vi "GUI_PiezoControllerMMC-100.vi"() -> ()   [LabVIEW 2013]
doc: "Example of using standard HTTP protocol for recieving a web site (the HTML source)\n\n\nThis example uses the GET command. For general information about the HTTP protocol and other commands go to\nhttp://www.w3.org/Protocols\n\n\nBjornar Svingen\nbjornar.svingen@sintef.no bjornar.svingen@ktv.no"
uses:
  Shared/GUI_Template/GUI_master/tcp_new_data_event.ctl
  Shared/GUI_Template/GUI_master/tcp new data cluster.ctl
  <vilib>/Utility/config.llb/NI_LVConfig.lvlib
  <vilib>/Utility/config.llb/Read Key (String).vi
panel:
  in  "Axis polarity::1":enum16{"default", "inverted"}(ring) caption="Axis polarity"
  in  "Deceleration::1":dbl caption="Deceleration (mm/s^2)" min=0.0 max=500.0
  in  "Acceleration::1":dbl caption="Acceleration (mm/s^2)" min=0.0 max=500.0
  in  "Velocity::1":dbl caption="Velocity (mm/s)" min=0.0 max=100.0
  in  "Home::1":enum16{"HOME", "POS (+)", "NEG (-)", "done"}(ring) caption="Homing"
  in  "EnableMotor::1":bool caption="Motor enable"
  out "Motor status::1":T1(ring) caption="Motor status"
  in  "Nloop enable::1":bool caption="N-loop enable"
  out "Encoder position::1":dbl caption="Encoder pos. (mm)" min=-13.0 max=13.0 format="%.6f"
  in  "position::1":dbl caption="Position (mm)" min=-13.0 max=13.0 format="%.6f"
  out "tcp data event 2":T2
  out "GUIdevice 1":string="HeatTL1Stage"
  in  "Exit":bool
  out "Error":T3
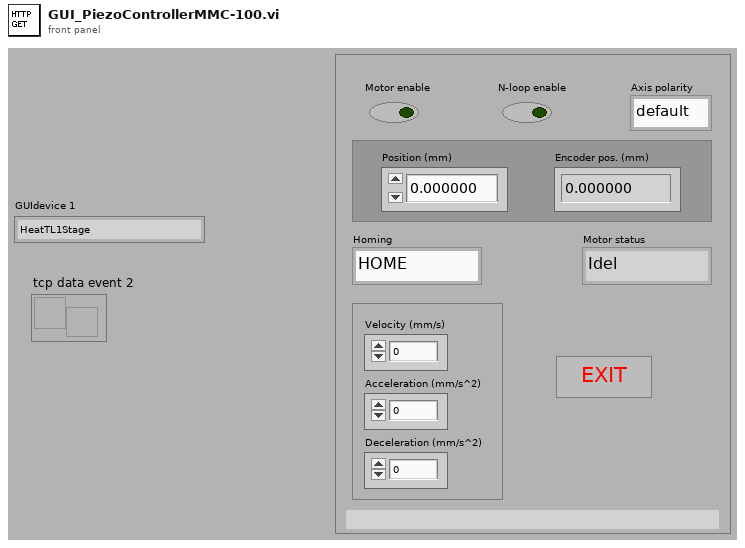
[diagram p1: front panel]
types:
  T1 = enum16{"Idel", "Moving", "Accelerating", "Decelerating", "L- (neg limit)", "L+ (pos limit)", "Homed", "Unknown"}
  T2 = typedef "tcp_new_data_event.ctl" = refnum<user-event>
  T3 = cluster{"status":bool, "code":i32, "UDP error message":string}
  T4 = enum32{"invalid app kind", "Development System", "Run Time System", "Student Edition", "Embedded LabVIEW", "Evaluation", "Custom"}
  T5 = typedef "tcp new data cluster.ctl" = cluster{"EventEnum":enum16{"new data", "connection status update"}, "Device name":string}
  T6 = enum32{"Invalid", "Standard", "Closed", "Hidden", "Minimized", "Maximized"}
  T7 = cluster{"Core":cluster{"Current VI Reference":refnum<vi>, "Close Panel on Exit?":bool}, "SuperGUI":cluster{"STOP queue":refnum<queue>, "SuperGUI ref":refnum<vi>, "event reg":refnum<event-registration>}, "Stage Device list":string[]}
  T8 = cluster{"STOP queue":refnum<queue>, "SuperGUI ref":refnum<vi>, "event reg":refnum<event-registration>}
  T9 = cluster{"Current VI Reference":refnum<vi>, "Close Panel on Exit?":bool}
  T10 = typedef "NI_LVConfig.lvlib/Config Data RefNum.ctl" = refnum<k1>
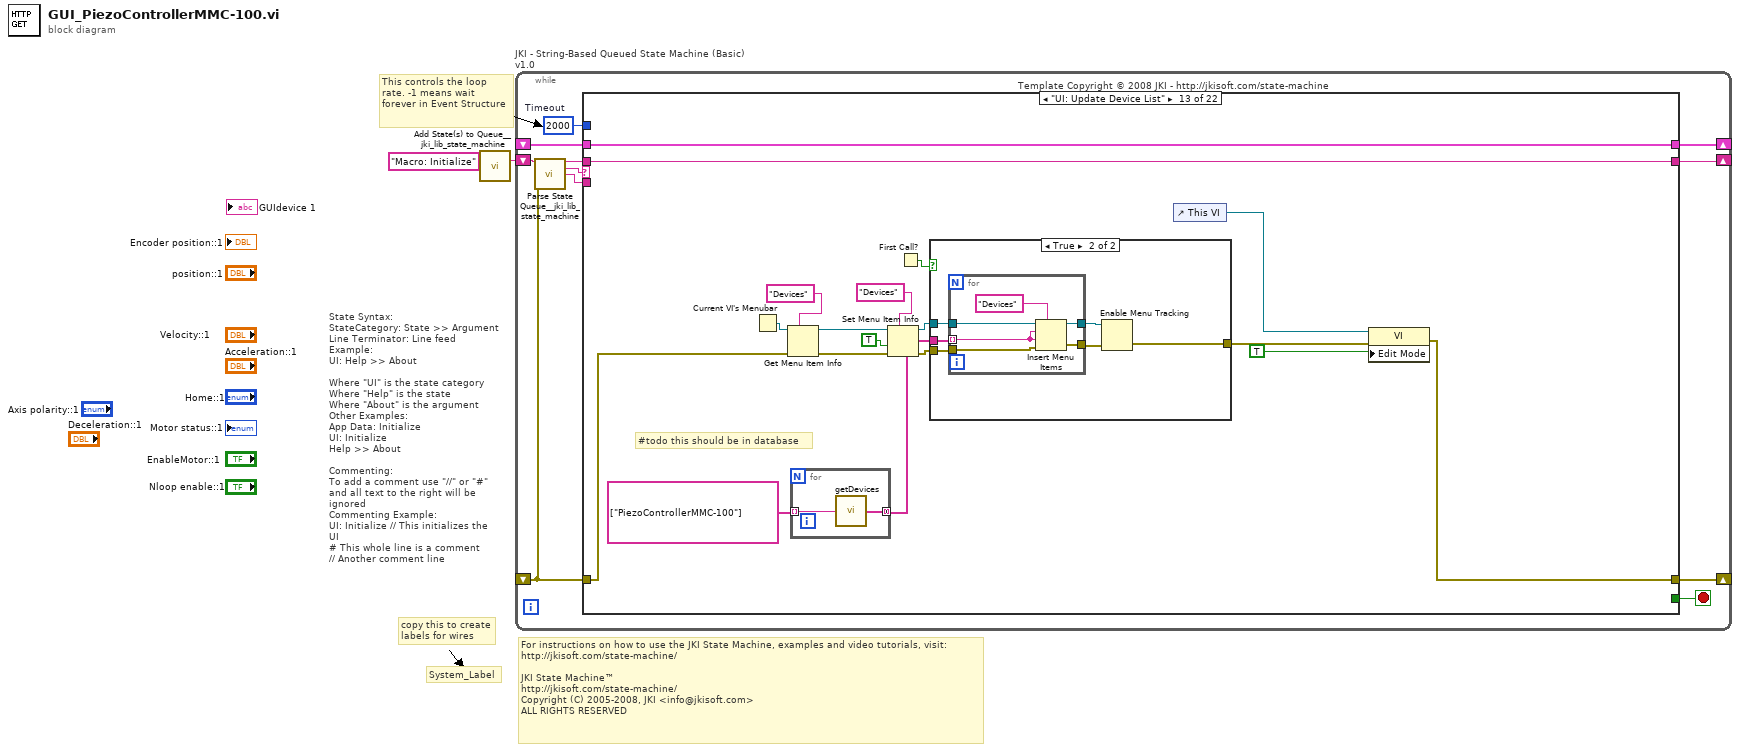
[diagram p0: block diagram]
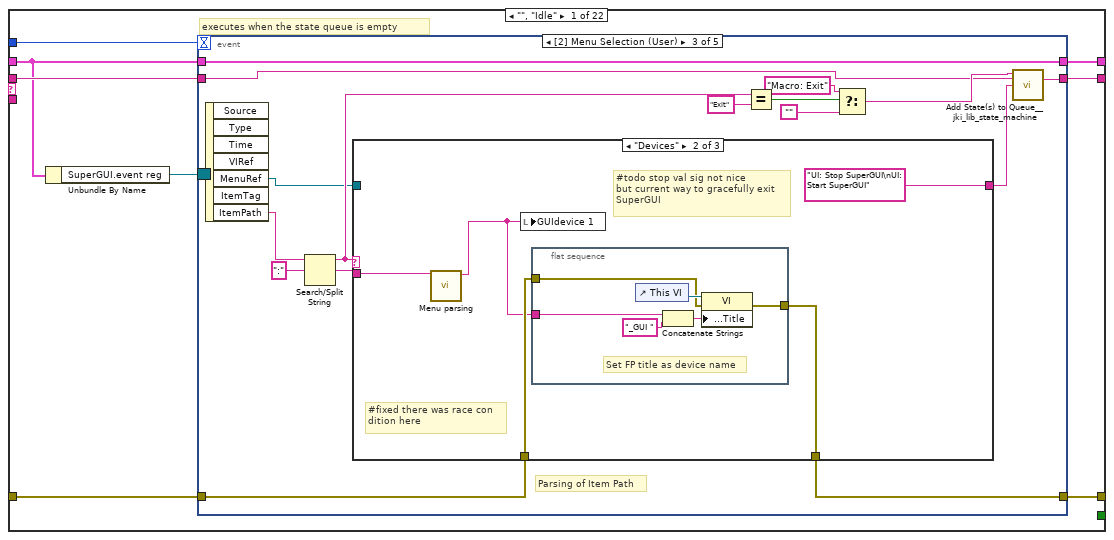
[diagram p2: hidden frame]
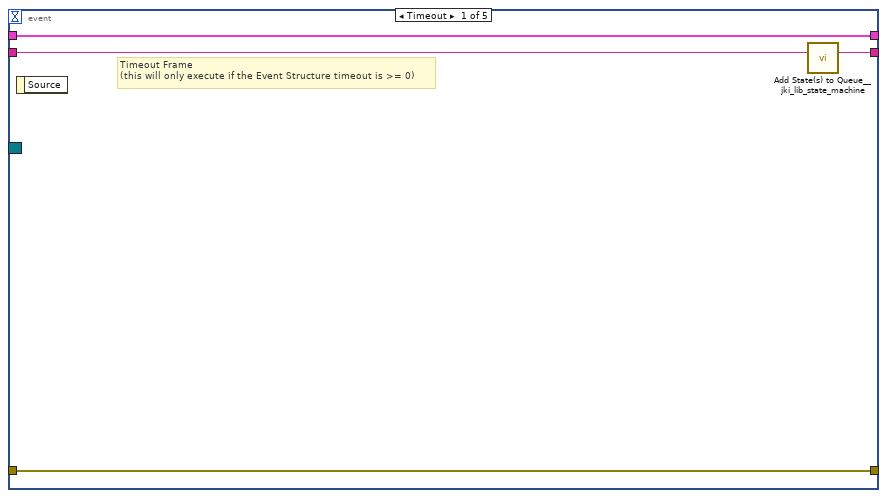
[diagram p3: hidden frame]
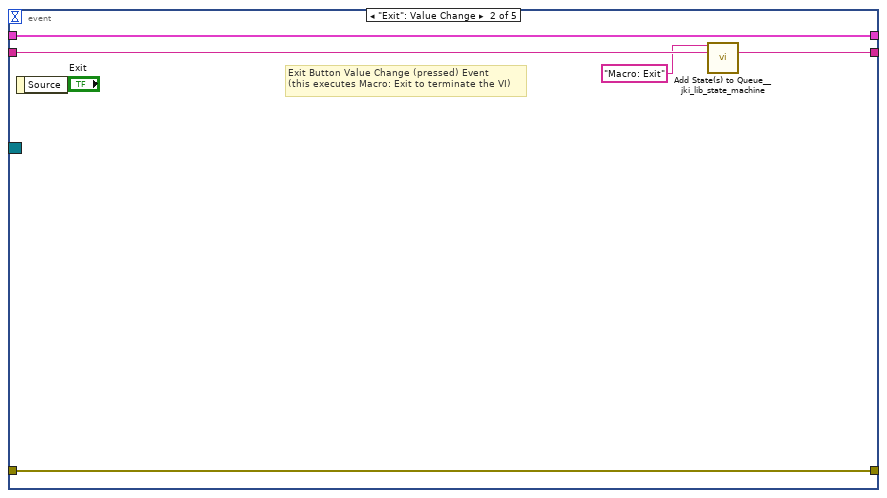
[diagram p4: hidden frame]
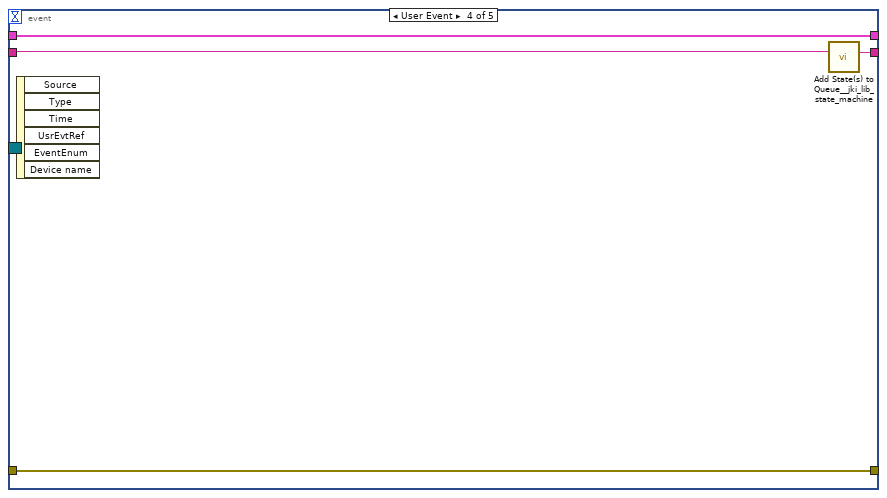
[diagram p7: hidden frame]
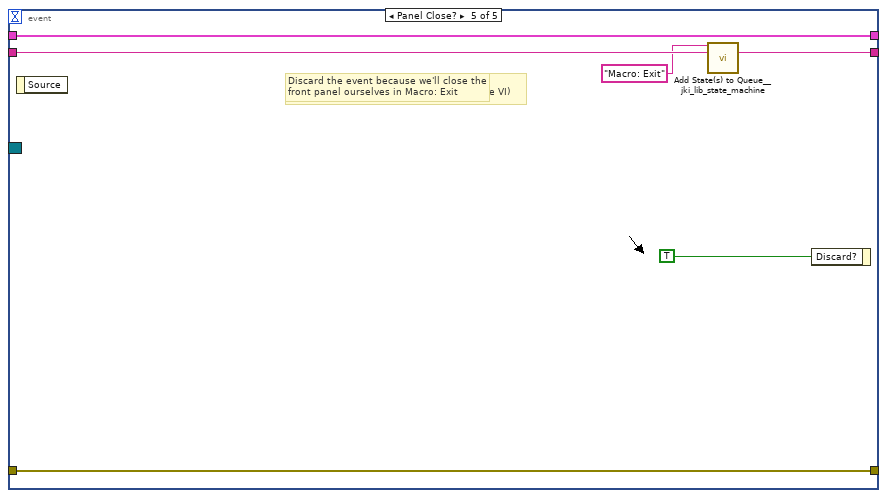
[diagram p8: hidden frame]
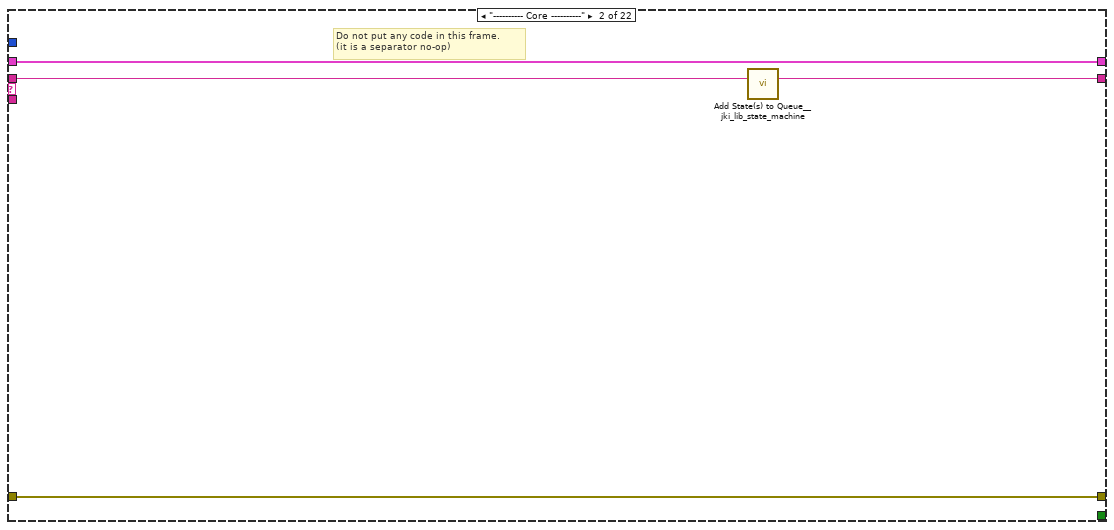
[diagram p9: hidden frame]
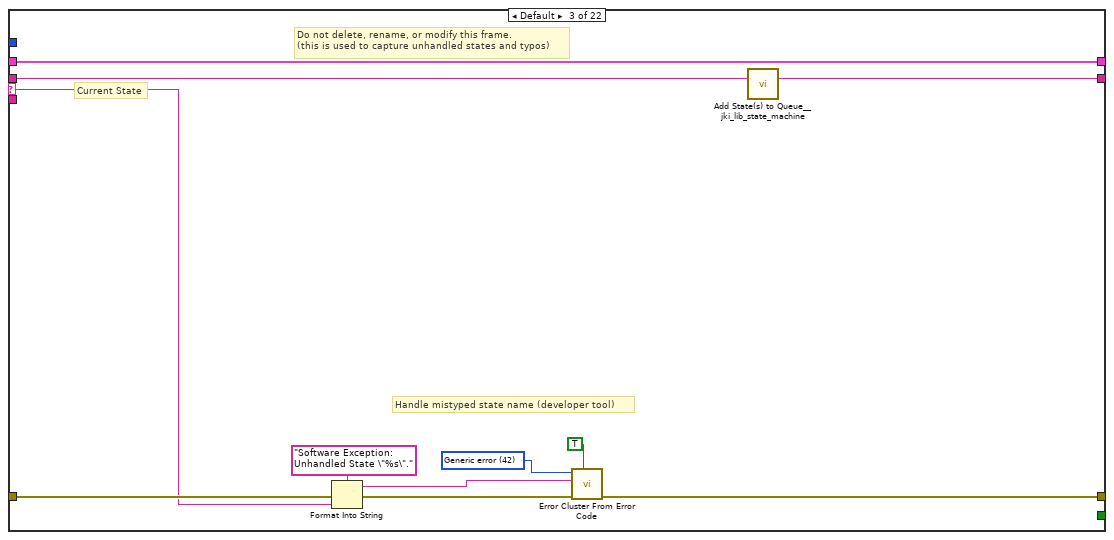
[diagram p10: hidden frame]
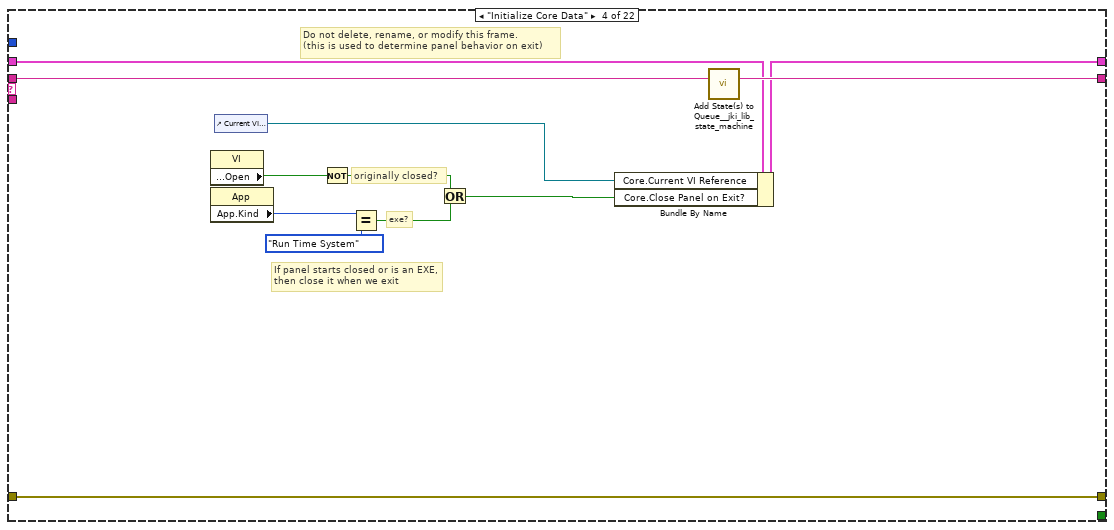
[diagram p11: hidden frame]
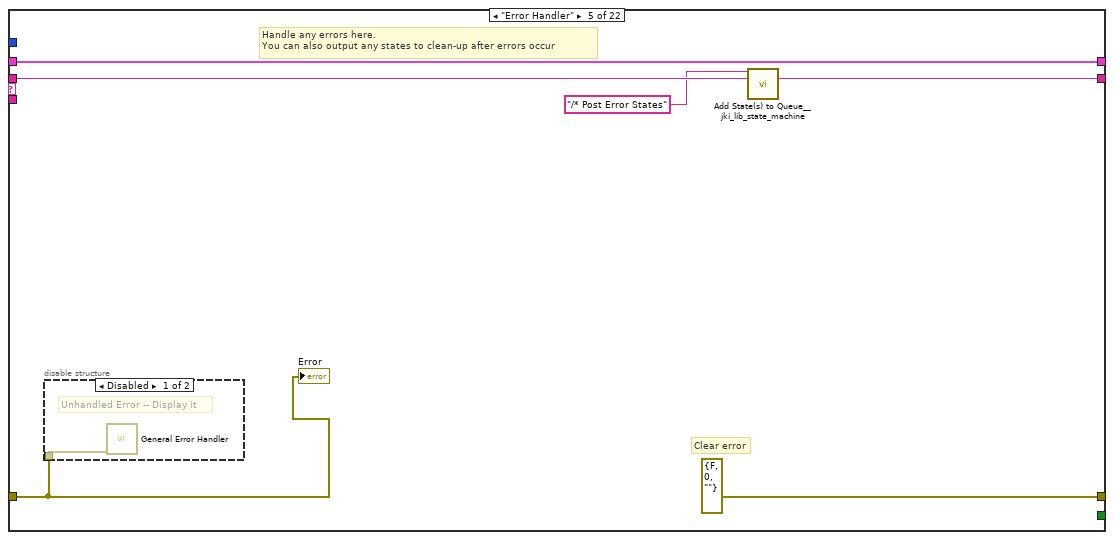
[diagram p12: hidden frame]
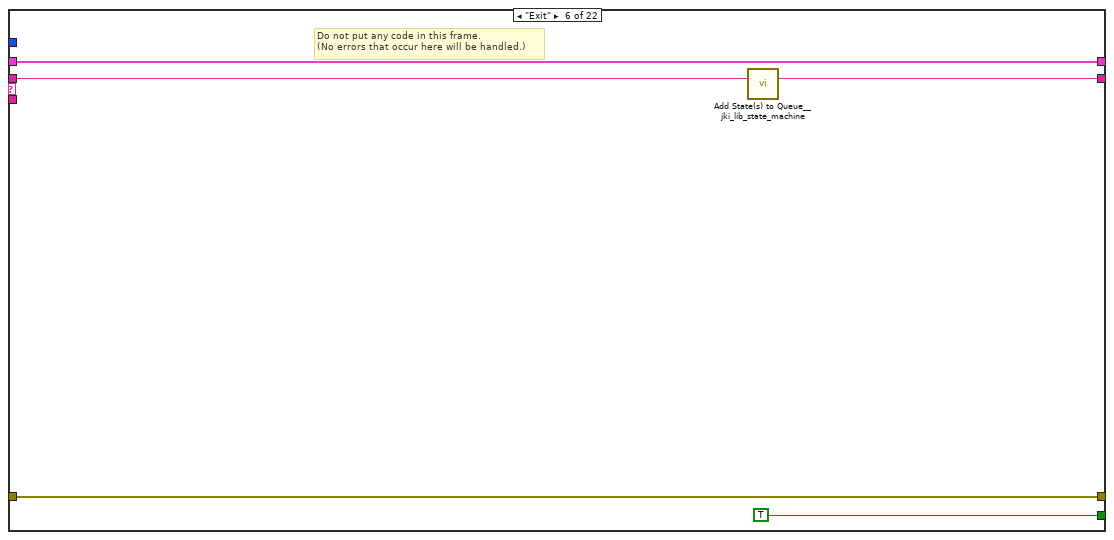
[diagram p14: hidden frame]
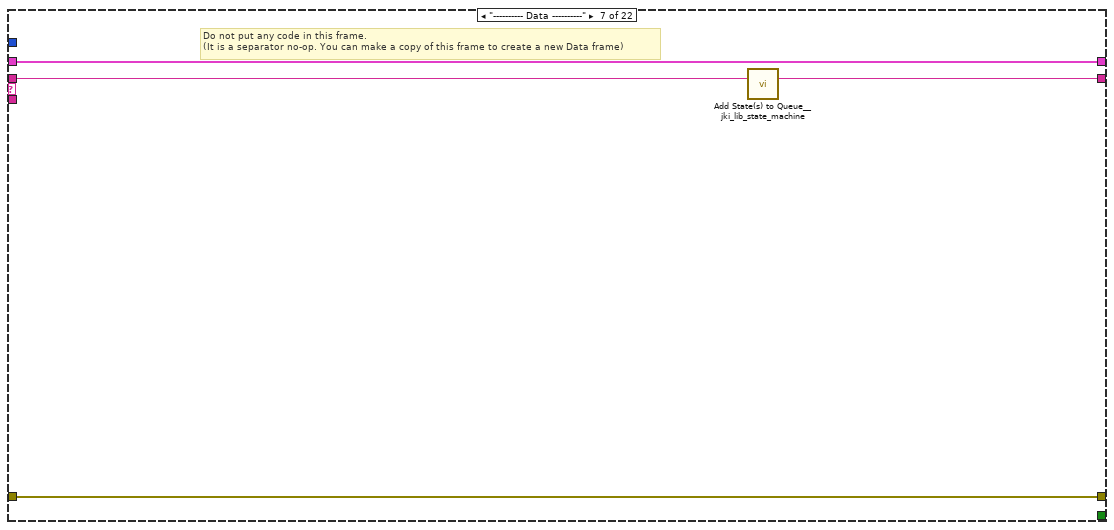
[diagram p15: hidden frame]
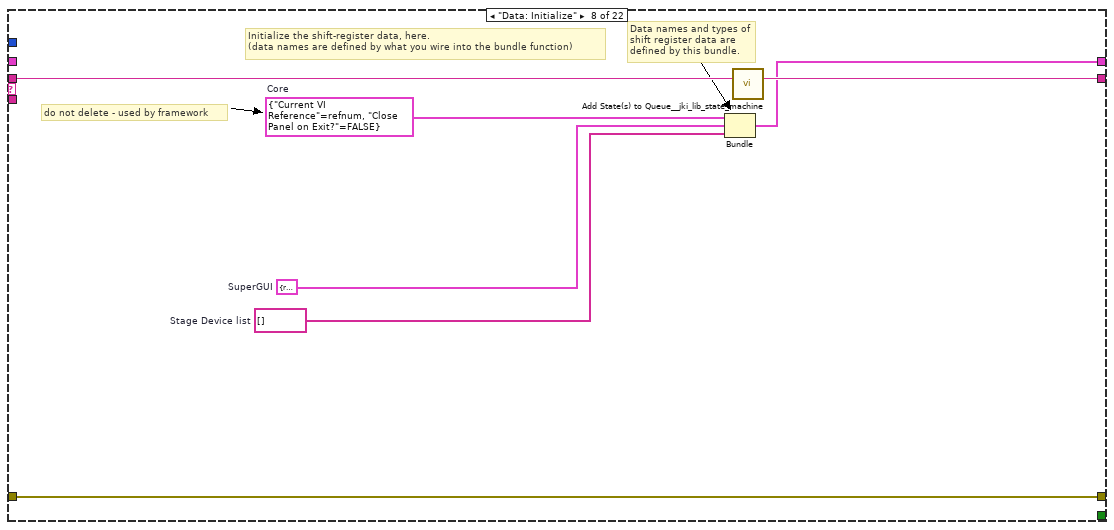
[diagram p16: hidden frame]
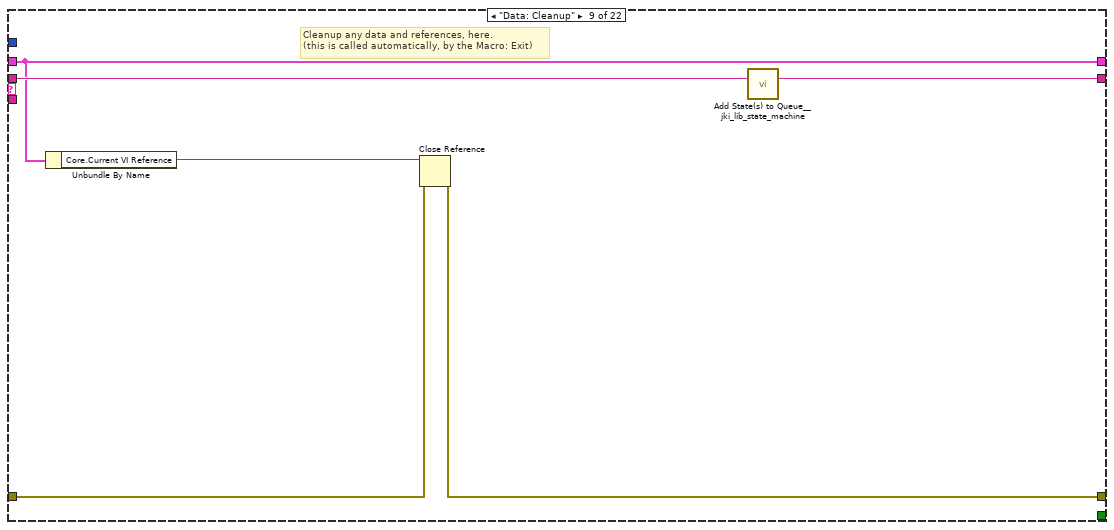
[diagram p17: hidden frame]
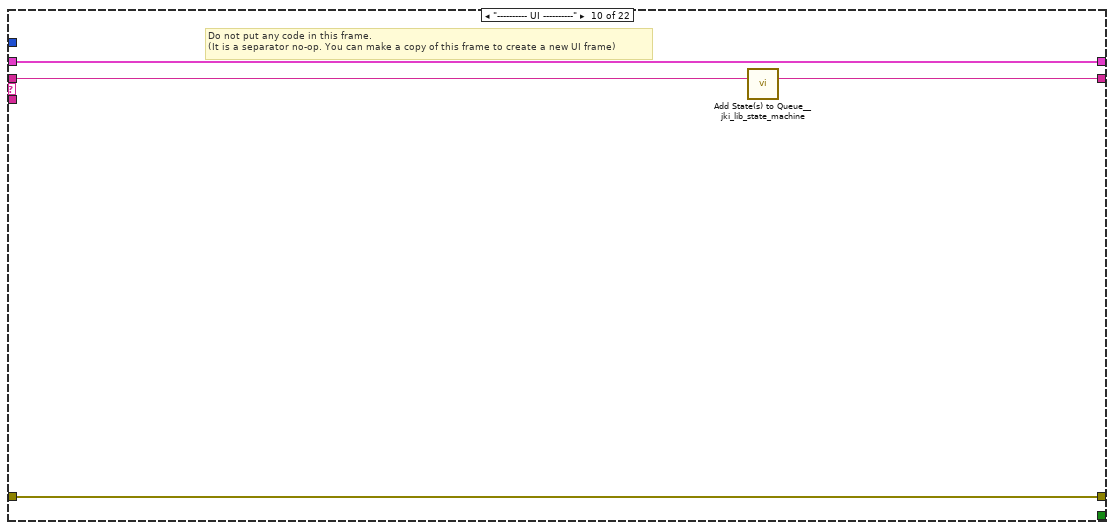
[diagram p18: hidden frame]
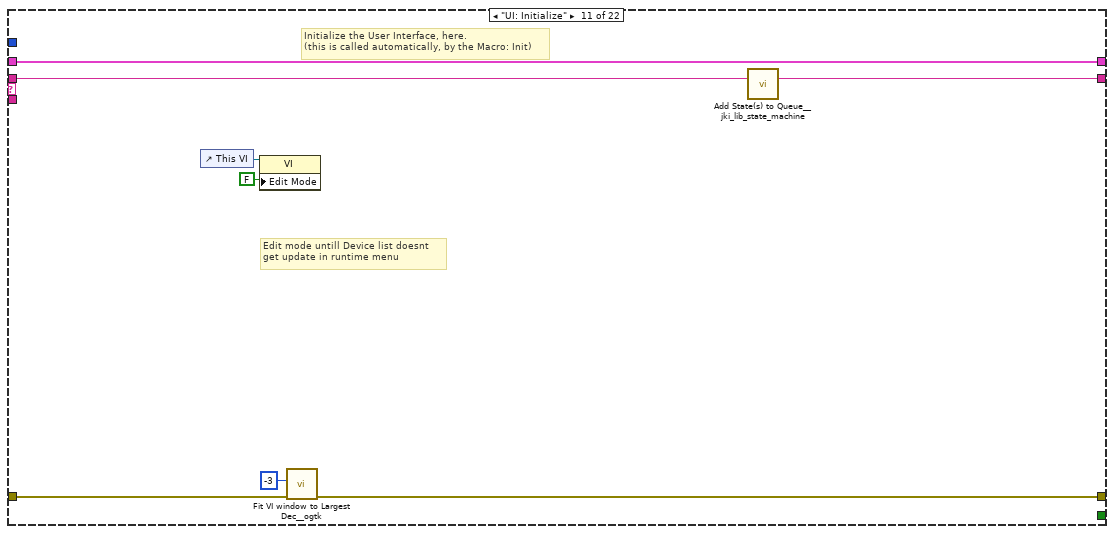
[diagram p19: hidden frame]
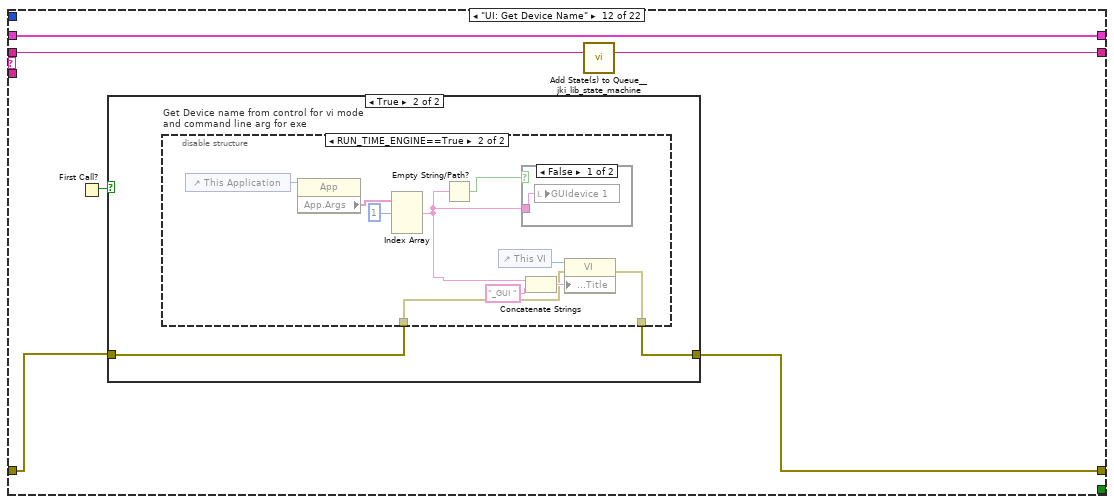
[diagram p20: hidden frame]
diagram:
  # "For instructions on how to use the JKI State Machine, examples and video tutorials, visit:\nhttp://jkisoft.com/state-machine/\n\nJKI State Machine™\nhttp://jkisoft.com/state-machine/\nCopyright (C) 2005-2008, JKI <info@jkisoft.com>\nALL RIGHTS RESERVED"
  # "State Syntax:\nStateCategory: State >> Argument\nLine Terminator: Line feed\nExample:\nUI: Help >> About\n\nWhere \"UI\" is the state category\nWhere \"Help\" is the state\nWhere \"About\" is the argument\nOther Examples:\nApp Data: Initialize\nUI: Initialize\nHelp >> About\n\nCommenting:\nTo add a comment use \"//\" or \"#\" and all text to the right will be ignored\nCommenting Example:\nUI: Initialize // This initializes the UI\n# This whole line is a comment\n// Another comment line"
  # "copy this to create labels for wires"
  # "This controls the loop rate. -1 means wait forever in Event Structure"
  # "System_Label"
  n1 = call <vilib>:"Add State(s) to Queue__jki_lib_state_machine.vi"("State(s) in (\"\")"="Macro: Initialize") -> ("States Out"=w2:string)  [unwired: 14 in]
  n2 = while "JKI - String-Based Queued State Machine (Basic) v1.0" {
    shift-right: [w6] -> _
    shift-left: _ -> [w5]
    shift-right: [w9] -> _
    shift-left: _ -> [w3]
    shift-right: [w8] -> _
    shift-left: w2 -> [w10]
    stop <- w7 stop-if-true
    w4 = 2000  # Timeout
    # "Template Copyright © 2008 JKI - http://jkisoft.com/state-machine"
    n3 = call <vilib>:"Parse State Queue__jki_lib_state_machine.vi"("State Queue"=w10, "Error In (no error)"=w3) -> ("Remaining States"=w12:string, "Current State"=w13:string, "Arguments"=w11:string)  [unwired: 11 in]
    n4 = case shown="\"UI: Update Device List\"" w13 {
      selector: w13 -> [_ _ w74 _ _ _ _ _ _ _ _ _ _ _ _ _ _ _ _ _ _ _]
      tunnel: w12 -> [w21 w73 w78 w96 w102 w108 w112 w119 w125 w129 w137 w139 w160 w199 w211 w224 w235 w261 w266 w276 w280 w284]
      tunnel: w11 -> [_ _ _ _ _ _ _ _ _ _ _ _ _ _ _ w219 w229 _ _ _ _ w282]
      tunnel: w5 -> [w15 w70 w76 w87 w99 w106 w109 _ w120 w126 w135 w138 w161 w196 w215 w222 w231 w258 w263 w273 w277 w285]
      tunnel: [w19 w71 w80 w93 errorcluster {"status"=FALSE, "code"=0, "source"=""} ("error out") w105 w110 w116 w121 w127 w133 w141 w162 w195 w213 w220 w232 w259 w264 w274 w278 w283] -> w9
      tunnel: w3 -> [w18 w71 w79 w93 w97 w105 w110 w116 w122 w127 w134 w142 w163 w194 w214 w221 w233 w259 w264 w274 w278 w281]
      tunnel: [w20 w72 w77 w95 w101 w107 w111 w118 w124 w128 w136 w140 w160 w198 w212 w223 w234 w260 w265 w275 w279 w284] -> w8
      tunnel: [_ _ _ _ _ TRUE _ _ _ _ _ _ _ _ _ _ _ _ _ _ _ _] -> w7
      tunnel: [w17 w70 w76 w94 w99 w106 w109 w117 w120 w126 w135 w138 w161 w197 w215 w222 w231 w258 w263 w273 w277 w285] -> w6
      tunnel: w4 -> [w16 _ _ _ _ _ _ _ _ _ _ _ _ _ _ _ _ _ _ _ _ _]
      frame "", "Idle" {
        # "executes when the state queue is empty"
        n5 = Unbundle By Name(w15) -> ("SuperGUI.event reg"=w14:refnum<event-registration>)
        n6 = event shown="[2] Menu Selection (User)" {
          selector: w14 -> [_ _ _ _ _]
          dyn-events: _ -> [_ _ _ _ _]
          timeout: w16 -> [_ _ _ _ _]
          tunnel: w21 -> [w25 w30 w34 w61 w69]
          tunnel: [w24 w29 w32 w62 w68] -> w20
          tunnel: w15 -> [w22 w27 w33 w60 w66]
          tunnel: [w23 w28 w38 w63 w67] -> w19
          tunnel: w18 -> [w23 w28 w37 w63 w67]
          tunnel: [w22 w27 w33 w60 w66] -> w17
          event Timeout {
            # "Timeout Frame\n(this will only execute if the Event Structure timeout is >= 0)"
            n7 = event-data() -> ()  [unwired: 1 in, 1 out]
            n8 = call <vilib>:"Add State(s) to Queue__jki_lib_state_machine.vi"("State(s) in (\"\")"=w25) -> ("States Out"=w24:string)  [unwired: 14 in]
          }
          event "Exit": Value Change {
            # "Exit Button Value Change (pressed) Event\n(this executes Macro: Exit to terminate the VI)"
            n9 = event-data() -> ()  [unwired: 1 in, 1 out]
            n10 = call <vilib>:"Add State(s) to Queue__jki_lib_state_machine.vi"("State(s) in Front (\"\")"="Macro: Exit", "State(s) in (\"\")"=w30) -> ("States Out"=w29:string)  [unwired: 13 in]
          }
          event Menu Selection (User) {
            # "Parsing of Item Path"
            n11 = event-data() -> ("MenuRef"=w36:refnum<k9>, "ItemPath"=w35:string)  [unwired: 1 in, 5 out]
            n12 = Search/Split String(string=w35, search string/char (-)=":") -> (substring before match=w45:string, match + rest of string=w39:string)  [unwired: 1 in, 1 out]
            n13 = case shown="\"Devices\"" w45 {
              tunnel: w39 -> [_ w52 _]
              tunnel: w36 -> [_ _ _]
              tunnel: w37 -> [w47 w51 w59]
              tunnel: [w47 w50 w59] -> w38
              tunnel: [_ "UI: Stop SuperGUI\nUI: Start SuperGUI" _] -> w46
              frame "", Default {
              }
              frame "Devices" {
                # "#fixed there was race con\ndition here"
                # "#todo stop val sig not nice\nbut current way to gracefully exit\nSuperGUI"
                n14 = call "Menu parsing.vi"("ItemPath"=w52) -> ("ItemPath"=w48:string)  [unwired: 9 in, 1 out]
                n15 = local write "GUIdevice 1"(w48) -> ()
                n16 = flat-sequence {
                  tunnel: [w55] -> w50
                  tunnel: w51 -> [w54]
                  tunnel: w48 -> [w53]
                  frame #0 {
                    # "Set FP title as device name"
                    n17 = control-ref of="This VI"() -> (w58:refnum<vi>)
                    n18 = Concatenate Strings(w53, "_GUI ") -> (w57:string)
                    n19 = property class="VI"(reference=w58, error in=w54, "Front Panel.Title"=w57) -> (error out=w55:errorcluster)  [unwired: 1 out]
                  }
                }
              }
              frame "Exit" {
              }
            }
            n20 = Equal?(x=w45, y="Exit") -> (x = y?=w41:bool)
            n21 = Select(t="Macro: Exit", s=w41, f="") -> (s? t:f=w44:string)
            n22 = call <vilib>:"Add State(s) to Queue__jki_lib_state_machine.vi"("State(s) in Front (\"\")"=w44, "State(s) in (\"\")"=w34, "State(s) at Back (\"\")"=w46) -> ("States Out"=w32:string)  [unwired: 12 in]
          }
          event User Event {
            n23 = event-data() -> ()  [unwired: 1 in, 6 out]
            n24 = call <vilib>:"Add State(s) to Queue__jki_lib_state_machine.vi"("State(s) in (\"\")"=w61) -> ("States Out"=w62:string)  [unwired: 14 in]
          }
          event Panel Close? {
            # "Discard the event because we'll close the front panel ourselves in Macro: Exit"
            # "Close Panel button (pressed) Event\n(this executes Macro: Exit to terminate the VI)"
            n25 = event-data() -> ()  [unwired: 1 in, 1 out]
            n26 = call <vilib>:"Add State(s) to Queue__jki_lib_state_machine.vi"("State(s) in Front (\"\")"="Macro: Exit", "State(s) in (\"\")"=w69) -> ("States Out"=w68:string)  [unwired: 13 in]
            n27 = event-data("Discard?"=TRUE) -> ()  [unwired: 1 in, 1 out]
          }
        }
      }
      frame "---------- Core ----------" {
        # "Do not put any code in this frame.\n(it is a separator no-op)"
        n28 = call <vilib>:"Add State(s) to Queue__jki_lib_state_machine.vi"("State(s) in (\"\")"=w73) -> ("States Out"=w72:string)  [unwired: 14 in]
      }
      frame Default {
        w83 = 42 items=["No error", "Argument error", "Memory is full", "Out of zone", "End of file", "File already open", "Generic file I/O error", "File not found", "File permission error", "Disk is full", "Duplicate path", "Too many files open", "System feature not enabled", "Resource file not found", "Cannot add resource", "Resource not found", "Image not found", "Image memory error", "Pen does not exist", "Config type invalid", "Config token not found", "Config parse error", "Config memory error", "Bad external code format", "Bad external code offset", "External code not present", "Null window", "Destroy window error", "Null menu", "Print aborted", "Bad print record", "Print driver error", "Windows error during printing", "Memory error during printing", "Print dialog error", "Generic print error", "Invalid device refnum", "Device not found", "Device parameter error", "Device unit error", "Cannot open device", "Device call aborted", "Generic error", "Cancelled by user", "Object ID too low", "Object ID too high", "Object not in heap", "Unknown heap", "Unknown object (invalid DefProc)", "Unknown object (DefProc not in table)", "Message out of range", "Invalid (null) method", "Unknown message", "Manager call not supported", "Bad address", "Network operation in progress", "Network operation timed out", "Connection is busy", "Network attribute not supported", "Network error", "Address in use", "System out of memory", "Connection aborted", "Connection refused", "Not connected", "Already connected", "Connection closed", "Initialization error (interapplication manager)", "Bad occurrence", "Wait on unbound occurrence handler", "Occurrence queue overflow", "Datalog type conflict", "Unused", "Unrecognized type (interapplication manager)", "Memory corrupt", "Failed to make temporary DLL", "Old CIN version", "Drag socket not found", "Failed to load drop-object", "Failed to register OLE object", "Failed to release OLE object", "Format specifier type mismatch", "Unknown format specifier", "Too few format specifiers", "Too many format specifiers", "Scan failed", "Newer CIN version", "Error converting to variant", "Runtime menu error", "Password tampered", "Variant attribute not found", "Incompatible variant data type", "Event data is not available", "Event Store is not present", "Occurrence is not found", "Event Queue is not created", "Event info is not available", "Refnum passed is NULL", "Error retrieving Class GUID", "Error retrieving CoClass GUID", "Error retrieving TypeLib GUID.", "Bad built application magic bytes.", "Specific driver is different from the specific driver associated with the Logical Name.", "There is no session opened to the class driver.", "Max Error", "MAX - Error with config objects", "MAX - Error loading configuration", "MAX - Group not supported"]
        # "Current State"
        # "Do not delete, rename, or modify this frame.\n(this is used to capture unhandled states and typos)"
        # "Handle mistyped state name (developer tool)"
        n29 = Format Into String(format string="Software Exception: Unhandled State \"%s\"." ("message"), error in=w79, w74) -> (resulting string=w82:string, error out=w81:errorcluster)  [unwired: 1 in]
        n30 = call <vilib>:"Error Cluster From Error Code.vi"("show call chain? (False)"=TRUE, "error in (no error)"=w81, "error message (\"\")"=w82, "error code (0)"=w83) -> ("error out"=w80:errorcluster)  [unwired: 5 in]
        n31 = call <vilib>:"Add State(s) to Queue__jki_lib_state_machine.vi"("State(s) in (\"\")"=w78) -> ("States Out"=w77:string)  [unwired: 14 in]
      }
      frame "Initialize Core Data" {
        # "Do not delete, rename, or modify this frame.\n(this is used to determine panel behavior on exit)"
        # "originally closed?"
        # "exe?"
        # "If panel starts closed or is an EXE, then close it when we exit"
        n32 = property class="VI"() -> ("Front Panel.Open"=w92:bool)  [unwired: 2 in, 2 out]
        n33 = property class="App"() -> ("App.Kind"=w91:T4)  [unwired: 2 in, 2 out]
        n34 = control-ref of="Current VI Reference"() -> (w85:refnum<vi>)
        n35 = Not(x=w92) -> (.not. x?=w89:bool)
        n36 = Equal?(x=w91, y=T4."Run Time System" ("Application:Kind")) -> (x = y?=w88:bool)
        n37 = Or(x=w89, y=w88) -> (x .or. y?=w86:bool)
        n38 = Bundle By Name(cluster=w87, "Core.Current VI Reference"=w85, "Core.Close Panel on Exit?"=w86) -> (w94:T7)
        n39 = call <vilib>:"Add State(s) to Queue__jki_lib_state_machine.vi"("State(s) in (\"\")"=w96) -> ("States Out"=w95:string)  [unwired: 14 in]
      }
      frame "Error Handler" {
        # "Handle any errors here.\nYou can also output any states to clean-up after errors occur"
        # "Clear error"
        n40 = disable-structure shown="Disabled" {
          disable-tunnel: w97 -> [w103 _]
          frame Disabled {
            # "Unhandled Error -- Display it"
            n41 = call <vilib>:"General Error Handler.vi"("error in (no error)"=w103) -> ()  [unwired: 10 in, 5 out]
          }
          frame Enabled {
          }
        }
        n42 = call <vilib>:"Add State(s) to Queue__jki_lib_state_machine.vi"("State(s) in Front (\"\")"="/* Post Error States", "State(s) in (\"\")"=w102) -> ("States Out"=w101:string)  [unwired: 13 in]
        "Error" <- w97
      }
      frame "Exit" {
        # "Do not put any code in this frame.\n(No errors that occur here will be handled.)"
        n43 = call <vilib>:"Add State(s) to Queue__jki_lib_state_machine.vi"("State(s) in (\"\")"=w108) -> ("States Out"=w107:string)  [unwired: 14 in]
      }
      frame "---------- Data ----------" {
        # "Do not put any code in this frame.\n(It is a separator no-op. You can make a copy of this frame to create a new Data frame)"
        n44 = call <vilib>:"Add State(s) to Queue__jki_lib_state_machine.vi"("State(s) in (\"\")"=w112) -> ("States Out"=w111:string)  [unwired: 14 in]
      }
      frame "Data: Initialize" {
        w113 = string[] []  # Stage Device list
        w114 = T8 {"STOP queue"=refnum, "SuperGUI ref"=refnum, "event reg"=refnum}  # SuperGUI
        w115 = T9 {"Current VI Reference"=refnum, "Close Panel on Exit?"=FALSE}  # Core
        # "do not delete - used by framework"
        # "Data names and types of shift register data are defined by this bundle."
        # "Initialize the shift-register data, here.\n(data names are defined by what you wire into the bundle function)"
        n45 = Bundle("Core"=w115, "SuperGUI"=w114, "Stage Device list"=w113) -> (w117:T7)  [unwired: 1 in]
        n46 = call <vilib>:"Add State(s) to Queue__jki_lib_state_machine.vi"("State(s) in (\"\")"=w119) -> ("States Out"=w118:string)  [unwired: 14 in]
      }
      frame "Data: Cleanup" {
        # "Cleanup any data and references, here.\n(this is called automatically, by the Macro: Exit)"
        n47 = Unbundle By Name(w120) -> ("Core.Current VI Reference"=w123:refnum<vi>)
        n48 = Close Reference(reference=w123, error in (no error)=w122) -> (error out=w121:errorcluster)
        n49 = call <vilib>:"Add State(s) to Queue__jki_lib_state_machine.vi"("State(s) in (\"\")"=w125) -> ("States Out"=w124:string)  [unwired: 14 in]
      }
      frame "---------- UI ----------" {
        # "Do not put any code in this frame.\n(It is a separator no-op. You can make a copy of this frame to create a new UI frame)"
        n50 = call <vilib>:"Add State(s) to Queue__jki_lib_state_machine.vi"("State(s) in (\"\")"=w129) -> ("States Out"=w128:string)  [unwired: 14 in]
      }
      frame "UI: Initialize" {
        # "Edit mode untill Device list doesnt \nget update in runtime menu"
        # "Initialize the User Interface, here.\n(this is called automatically, by the Macro: Init)"
        n51 = control-ref of="This VI"() -> (w131:refnum<vi>)
        n52 = property class="VI"(reference=w131, "Edit Mode"=FALSE ("Edit Mode On Open")) -> ()  [unwired: 1 in, 2 out]
        n53 = call <userlib>:"Fit VI window to Largest Dec__ogtk.vi"("error in (no error)"=w134, "border spacing (2 px)"=-3) -> ("error out"=w133:errorcluster)  [unwired: 4 in, 1 out]
        n54 = call <vilib>:"Add State(s) to Queue__jki_lib_state_machine.vi"("State(s) in (\"\")"=w137) -> ("States Out"=w136:string)  [unwired: 14 in]
      }
      frame "UI: Get Device Name" {
        n55 = First Call?() -> (First Call?: T/F=w143:bool)
        n56 = case shown="True" w143 {
          tunnel: w142 -> [w144 w146]
          tunnel: [w144 w145] -> w141
          frame False {
          }
          frame True {
            n57 = disable-structure "Get Device name from control for vi mode\nand command line arg for exe" shown="RUN_TIME_ENGINE==True" {
              disable-tunnel: w146 -> [_ w148]
              disable-tunnel: [_ w147] -> w145
              frame condition #0 (active) {
              }
              frame condition #1 {
                n58 = control-ref of="This Application"() -> (w156:refnum<vi>)
                n59 = property class="App"(reference=w156) -> ("App.Args"=w155:string[])  [unwired: 1 in, 2 out]
                n60 = Index Array(array=w155, index #1=1 ("index")) -> (element #1=w149:string)  [unwired: 2 in, 2 out]
                n61 = Empty String/Path?(string/path=w149) -> (empty?=w153:bool)
                n62 = control-ref of="This VI"() -> (w152:refnum<vi>)
                n63 = case shown="False" w153 {
                  tunnel: w149 -> [w157 _]
                  frame False {
                    n64 = local write "GUIdevice 1"(w157) -> ()
                  }
                  frame True {
                  }
                }
                n65 = Concatenate Strings(w149, "_GUI ") -> (w151:string)
                n66 = property class="VI"(reference=w152, error in=w148, "Front Panel.Title"=w151) -> (error out=w147:errorcluster)  [unwired: 1 out]
              }
            }
          }
        }
        n67 = call <vilib>:"Add State(s) to Queue__jki_lib_state_machine.vi"("State(s) in (\"\")"=w139) -> ("States Out"=w140:string)  [unwired: 14 in]
      }
      frame "UI: Update Device List" {
        # "#todo this should be in database"
        n68 = Current VI's Menubar() -> (w173:refnum<k9>)
        n69 = Get Menu Item Info(7:"Devices" ("item tag"), 8:w163, 11:w173) -> (0:w166:errorcluster, 3:w171:refnum<k9>)  [unwired: 5 out]
        n70 = for {
          tunnel: [w177] -> w158 mode=concatenating
          tunnel: string[] ["PiezoControllerMMC-100"] -> [w176] mode=indexing
          n71 = call "getDevices.vi"("Device Class"=w176) -> ("All Devices"=w177:string[])
        }
        n72 = Set Menu Item Info(7:"Devices" ("item tag"), 8:w166, 9:TRUE ("enabled"), 11:w171) -> (0:w167:errorcluster, 3:w169:refnum<k9>)  [unwired: 3 in]
        n73 = First Call?() -> (First Call?: T/F=w175:bool)
        n74 = case shown="True" w175 {
          tunnel: w169 -> [_ w183]
          tunnel: w158 -> [_ w182]
          tunnel: w167 -> [w178 w180]
          tunnel: [w178 w179] -> w165
          frame False {
          }
          frame True {
            n75 = for {
              tunnel: [w190] -> w184
              tunnel: w182 -> [w188] mode=indexing
              tunnel: w183 -> [w187]
              tunnel: [w186] -> w181
              tunnel: w180 -> [w185]
              n76 = Insert Menu Items(5:"Devices" ("menu tag"), 6:w185, 7:w188, 8:w188, 9:w187) -> (0:w186:errorcluster, 3:w190:refnum<k9>)  [unwired: 1 in, 1 out]
            }
            n77 = Enable Menu Tracking(2:w181, 4:w184) -> (0:w179:errorcluster)  [unwired: 1 in, 1 out]
          }
        }
        n78 = control-ref of="This VI"() -> (w164:refnum<vi>)
        n79 = property class="VI"(reference=w164, error in=w165, "Edit Mode"=TRUE ("Edit Mode On Open")) -> (error out=w162:errorcluster)  [unwired: 1 out]
      }
      frame "UI: Start SuperGUI" {
        # "create stop queue for supergui and its clones"
        # "x100 abort will be dependent on caller VI\nx80 abort will be independent of caller vi, this will abort vi when labview is closed."
        n80 = vi-ref "GUI_Master_subvi_reentrant_queues.vi"() -> (w202:refnum<vi>)
        n81 = Create User Event(user event datatype=T5 {"EventEnum"=enum."new data", "Device name"="Device name"} ("New Event")) -> (user event=w192:refnum<user-event>)  [unwired: 1 in, 1 out]
        "tcp data event 2" <- w192
        n82 = register-events(w192) -> (reference out=w191:refnum<event-registration>)  [unwired: 2 in, 1 out]
        n83 = property class="VI"(reference=w202) -> ("Path"=w201:path)  [unwired: 1 in, 2 out]
        n84 = control-ref of="This Application"() -> (w205:refnum<vi>)
        n85 = control-ref of="This VI"() -> (w204:refnum<vi>)
        n86 = Open VI Reference(type specifier VI Refnum (for type only)=refnum<vi> refnum, vi path=w201, options=256) -> (vi reference=w210:refnum<vi>, error out=w209:errorcluster)  [unwired: 3 in]
        n87 = call "supergui create stop queue.vi"() -> ("STOP Queue out"=w206:refnum<queue>)  [unwired: 11 in]
        n88 = Current VI's Menubar() -> (w203:refnum<k9>)
        n89 = call-by-ref "Start Asynchronous Call"(reference=w210, error in=w209, "STOP Queue in"=w206, "This Application"=w205, 8:"error in (no error)"=w194, "tcp data event"=w192, "Caller menu reference"=w203, "Caller VI ref"=w204) -> (reference out=w200:refnum<vi>, error out=w195:errorcluster)  [unwired: 5 in, 1 out]
        n90 = Bundle By Name(cluster=w196, "SuperGUI.event reg"=w191, "SuperGUI.SuperGUI ref"=w200, "SuperGUI.STOP queue"=w206) -> (w197:T7)
        n91 = call <vilib>:"Add State(s) to Queue__jki_lib_state_machine.vi"("State(s) in (\"\")"=w199) -> ("States Out"=w198:string)  [unwired: 14 in]
      }
      frame "UI: Stop SuperGUI" {
        n92 = Unbundle By Name(w215) -> ("SuperGUI.SuperGUI ref"=w217:refnum<vi>, "SuperGUI.STOP queue"=w216:refnum<queue>)
        n93 = Release Queue(queue=w216, error in (no error)=w214) -> (error out=w218:errorcluster)  [unwired: 1 in, 2 out]
        n94 = call-by-ref "Wait On Asynchronous Call"(reference=w217, error in=w218) -> ("error out"=w213:errorcluster)  [unwired: 11 in, 2 out]
        n95 = call <vilib>:"Add State(s) to Queue__jki_lib_state_machine.vi"("State(s) in (\"\")"=w211) -> ("States Out"=w212:string)  [unwired: 14 in]
      }
      frame "UI: Cursor Set" {
        # "Argument"
        # "Set and Unset Cursor Busy.\n(Usage: \"UI: Cursor Set >> Busy|Idle\")"
        n96 = case shown="\"Idle\", Default" w219 {
          tunnel: w221 -> [w226 w228]
          tunnel: [w225 w227] -> w220
          frame "Idle", Default {
            n97 = call <vilib>:"Unset Busy.vi"("error in (no error)"=w226) -> ("error out"=w225:errorcluster)  [unwired: 10 in]
          }
          frame "Busy" {
            n98 = call <vilib>:"Set Busy.vi"("error in (no error)"=w228) -> ("error out"=w227:errorcluster)  [unwired: 9 in, 1 out]
          }
        }
        n99 = call <vilib>:"Add State(s) to Queue__jki_lib_state_machine.vi"("State(s) in (\"\")"=w224) -> ("States Out"=w223:string)  [unwired: 14 in]
      }
      frame "UI: Front Panel State" {
        # "Argument"
        # "Set Front Panel Open or Closed\n(Usage: \"UI: Front Panel State >> Open|Close\")"
        n100 = Unbundle By Name(w231) -> ("Core.Current VI Reference"=w230:refnum<vi>)
        n101 = case shown="\"Open\", Default" w229 {
          tunnel: w233 -> [w239 w252]
          tunnel: [w241 w253] -> w232
          tunnel: w230 -> [w240 w250]
          frame "Open", Default {
            n102 = property class="VI"(reference=w240, error in=w239) -> (reference out=w237:refnum<vi>, error out=w238:errorcluster, "Front Panel.Open"=w236:bool)
            n103 = case shown="False" w236 {
              tunnel: [w244 w247] -> w241
              tunnel: w238 -> [w243 w247]
              tunnel: w237 -> [w242 _]
              frame False {
                n104 = invoke class="VI" method="FP.Open"(reference=w242, error in=w243, "Activate"=TRUE, "State"=T6."Standard") -> (error out=w244:errorcluster)  [unwired: 1 in, 4 out]
              }
              frame True {
              }
            }
          }
          frame "Close" {
            n105 = property class="VI"(reference=w250, error in=w252) -> (reference out=w249:refnum<vi>, error out=w251:errorcluster, "Front Panel.Open"=w248:bool)
            n106 = case shown="True" w248 {
              tunnel: [w254 w257] -> w253
              tunnel: w251 -> [w254 w256]
              tunnel: w249 -> [_ w255]
              frame False {
              }
              frame True {
                n107 = invoke class="VI" method="FP.Close"(reference=w255, error in=w256) -> (error out=w257:errorcluster)  [unwired: 1 in, 2 out]
              }
            }
          }
        }
        n108 = call <vilib>:"Add State(s) to Queue__jki_lib_state_machine.vi"("State(s) in (\"\")"=w235) -> ("States Out"=w234:string)  [unwired: 14 in]
      }
      frame "---------- Macro ----------" {
        # "Do not put any code in this frame.\n(It is a separator no-op. You can make a copy of this frame to create a new Macro frame)"
        n109 = call <vilib>:"Add State(s) to Queue__jki_lib_state_machine.vi"("State(s) in (\"\")"=w261) -> ("States Out"=w260:string)  [unwired: 14 in]
      }
      frame "Macro: Initialize" {
        w262 = "Data: Initialize\nInitialize Core Data\nUI: Initialize\nUI: Get Device Name\nUI: Update Device List\nUI: Start SuperGUI\nUI: Front Panel State >> Open"  # Data: Initialize Initialize Core Data UI: Initialize UI: Get Device Name UI: Update Device List UI: Start SuperGUI UI: Front Panel State >> Open
        # "Initialization Macro\n(This is called once, when the VI starts)"
        n110 = call <vilib>:"Add State(s) to Queue__jki_lib_state_machine.vi"("State(s) in Front (\"\")"=w262, "State(s) in (\"\")"=w266) -> ("States Out"=w265:string)  [unwired: 13 in]
      }
      frame "Macro: Exit" {
        # "Exit Macro\n(This is called once, when the VI exits)"
        n111 = Unbundle By Name(w273) -> ("Core.Close Panel on Exit?"=w272:bool)
        n112 = Select(t="UI: Front Panel State >> Close", s=w272, f="") -> (s? t:f=w269:string)
        n113 = call <vilib>:"Add State(s) to Queue__jki_lib_state_machine.vi"("State(s) in (\"\")"=w269, "State(s) at Back (\"\")"="Data: Cleanup\nExit") -> ("States Out"=w267:string)  [unwired: 13 in]
        n114 = call <vilib>:"Add State(s) to Queue__jki_lib_state_machine.vi"("State(s) in Front (\"\")"=w267, "State(s) in (\"\")"=w276) -> ("States Out"=w275:string)  [unwired: 13 in]
      }
      frame "---------- New Category ----------" {
        # "Template Separator\n(You can make a copy of, or modify, this frame)"
        n115 = call <vilib>:"Add State(s) to Queue__jki_lib_state_machine.vi"("State(s) in (\"\")"=w280) -> ("States Out"=w279:string)  [unwired: 14 in]
      }
      frame "action: read .txt" {
        n116 = disable-structure shown="Disabled" {
          disable-tunnel: [w292 w313] -> w283
          disable-tunnel: w282 -> [w289 _]
          disable-tunnel: w281 -> [w288 w313]
          frame Disabled {
            n117 = call "get software root directory.vi"() -> ("Application Directory"=w297:path)  [unwired: 11 in]
            n118 = Strip Path(path=w297) -> (stripped path=w296:path)  [unwired: 1 out]
            n119 = Build Path(base path=w296, name or relative path="user data\\Avocent_PSU_Labels.txt") -> (appended path=w295:path)
            n120 = property on="GUIdevice 1" class="Str"(error in=w288) -> (error out=w287:errorcluster, "Value"=w286:string)  [unwired: 1 in, 1 out]
            n121 = call <vilib>:"Open Config Data.vi"("error in (no error)"=w287, "create file if necessary (T)"=FALSE, "configuration file path"=w295) -> ("error out"=w293:errorcluster, "refnum"=w294:T10)  [unwired: 6 in, 1 out]
            n122 = for {
              N: 16 -> [_]
              tunnel: w294 -> [w311]
              tunnel: w293 -> [w310]
              tunnel: [w309] -> w292
              tunnel: [w308] -> w291 mode=indexing
              tunnel: w286 -> [w301]
              i -> [w303]
              n123 = Add(x=w303, y=1) -> (x+y=w304:i32)
              n124 = Number To Decimal String(number=w304) -> (decimal integer string=w306:string)  [unwired: 1 in]
              n125 = Concatenate Strings("Label " ("key"), w306) -> (w305:string)
              n126 = call-poly <vilib>:"Read Key.vi"("section"=w301, "error in (no error)"=w310, "default value"="", "key"=w305, "refnum"=w311) -> ("error out"=w309:errorcluster, "value"=w308:string)  [unwired: 3 in, 2 out]
            }
            n127 = case shown="Default" w289 {
              tunnel: w291 -> [w300 _]
              frame "av1" {
              }
              frame Default {
              }
            }
          }
          frame Enabled {
          }
        }
      }
    }
  }
